vi "ABAPI Dist Boolean to (0,2).vi"(4 "Boolean":bool) -> (1 "0, 2":u8)   [LabVIEW 2020]
doc: "This VI will convert a Boolean input to a numeric 0 or 2. If the Boolean is true a 2 is returned, if it is false a 0 is returned. This is useful for wiring up to the disabled attribute node to make a control or indicator either enabled (0) or disabled and grayed out (2)."
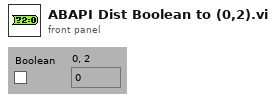
[diagram p1: front panel]
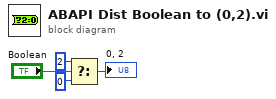
[diagram p0: block diagram]
diagram:
  n1 = Select(t=u8 2 ("y"), s="Boolean", f=u8 0 ("y")) -> (s? t:f=→"0, 2":u8)
